vi "test Basic Error Resolution.vi"(8 "error in (no error)":errorcluster, 11 "TestCase in":refnum<class "Task Tests.lvclass">) -> (0 "error out":errorcluster, 3 "TestCase out":refnum<class "Task Tests.lvclass">)   [LabVIEW 2017, in "Task Tests.lvclass"]
uses:
  Task Tests.lvclass
  <vilib>/Utility/error.llb/Error Cluster From Error Code.vi
  <vilib>/ErrorRing/Error Ring.xnode
  <vilib>/addons/_JKI Toolkits/VI Tester/TestCase.llb/TestCase.lvclass
  Futures/Task/Task.lvclass
  C:/Program Files (x86)/National Instruments/LabVIEW 2017/vi.lib/addons/_JKI Toolkits/VI Tester/TestCase.llb/TestCase.lvclass
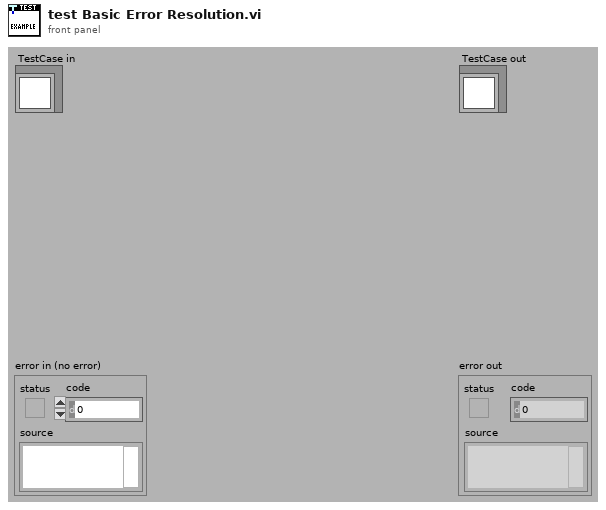
[diagram p1: front panel]
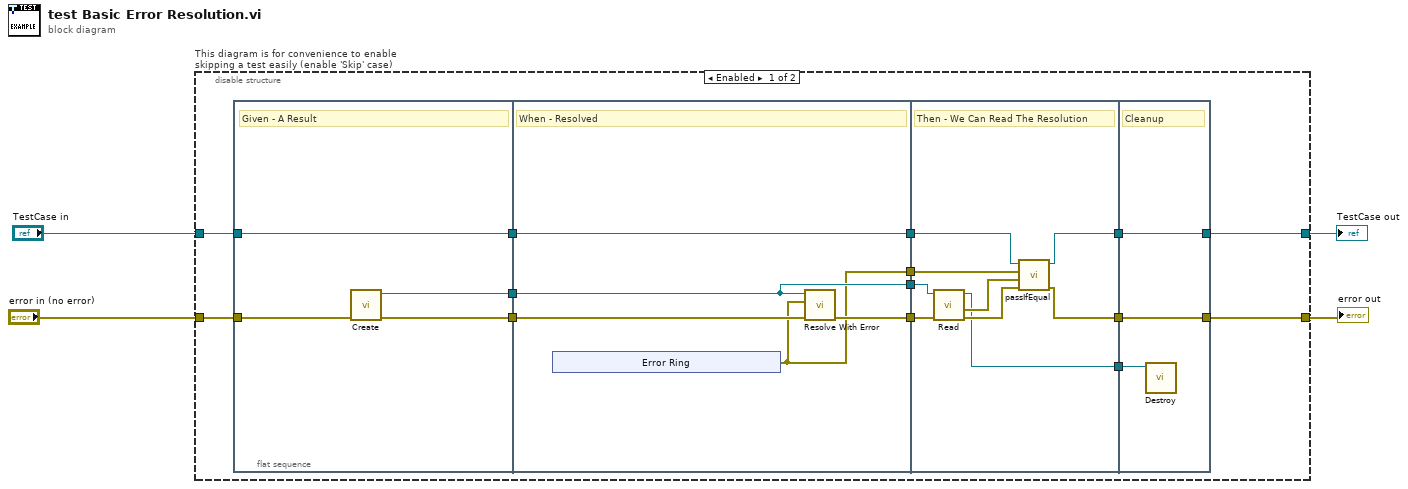
[diagram p0: block diagram]
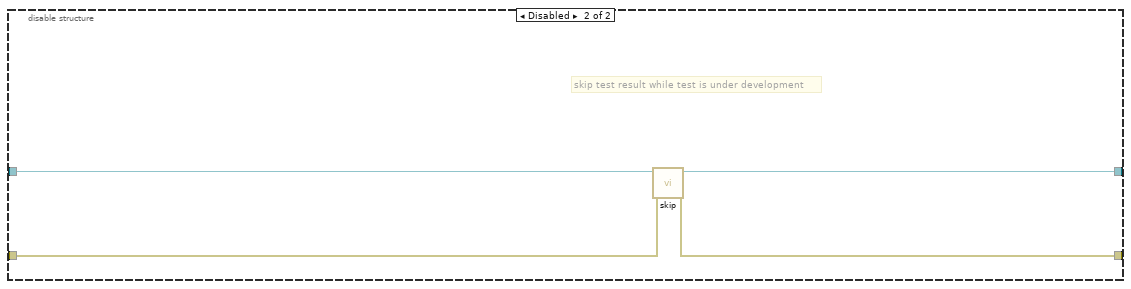
[diagram p2: hidden frame]
diagram:
  n1 = disable-structure "This diagram is for convenience to enable skipping a test easily (enable 'Skip' case)" shown="Enabled" {
    disable-tunnel: "TestCase in" -> [w12 w47]
    disable-tunnel: [w10 w45] -> w1
    disable-tunnel: [w9 w46] -> w3
    disable-tunnel: "error in (no error)" -> [w11 w44]
    frame Enabled {
      n2 = flat-sequence {
        tunnel: w11 -> [w21]
        tunnel: w12 -> [w22]
        tunnel: [w22] -> w18
        tunnel: [w20] -> w17
        tunnel: [w19] -> w8
        tunnel: [w27] -> w16
        tunnel: [w25] -> w15
        tunnel: w18 -> [w27]
        tunnel: w17 -> [w26]
        tunnel: w8 -> [w24]
        tunnel: [w24] -> w7
        tunnel: [w23] -> w6
        tunnel: [w39] -> w14
        tunnel: [w38] -> w13
        tunnel: w16 -> [w40]
        tunnel: w15 -> [w37]
        tunnel: w7 -> [w36]
        tunnel: w6 -> [w35]
        tunnel: [w32] -> w5
        tunnel: [w42] -> w9
        tunnel: [w43] -> w10
        tunnel: w14 -> [w43]
        tunnel: w13 -> [w42]
        tunnel: w5 -> [w41]
        frame #0 {
          # "Given - A Result"
          n3 = call "Create.vi"("error in (no error)"=w21) -> ("error out"=w20:errorcluster, "Result out"=w19:refnum<class "Task.lvclass">)  [unwired: 9 in]
        }
        frame #1 {
          # "When - Resolved"
          n4 = xnode "Error Ring"() -> ("error out"=w23:errorcluster)
          n5 = call "Resolve With Error.vi"("error in (no error)"=w26, "Error"=w23, "Result in"=w24) -> ("error out"=w25:errorcluster)  [unwired: 8 in]
        }
        frame #2 {
          # "Then - We Can Read The Resolution"
          n6 = call "Read.vi"("error in (no error)"=w37, "Result in"=w36) -> ("error out"=w34:errorcluster, "result error"=w33:errorcluster, "Result Out"=w32:refnum<class "Task.lvclass">)  [unwired: 5 in, 2 out]
          n7 = call-dynamic "passIfEqual.vi"("error in (no error)"=w34, "y"=w33, "x"=w35, "TestCase in"=w40) -> ("error out"=w38:errorcluster, "TestCase out"=w39:refnum<class "Task Tests.lvclass">)  [unwired: 6 in]
        }
        frame #3 {
          # "Cleanup"
          n8 = call "Destroy.vi"("Result in"=w41) -> ()  [unwired: 10 in, 1 out]
        }
      }
    }
    frame Disabled {
      # "skip test result while test is under development"
      n9 = call <vilib>:"skip.vi"("error in (no error)"=w44, "TestCase in"=w47) -> ("error out"=w46:errorcluster, "TestCase out"=w45:refnum<class "Task Tests.lvclass">)  [unwired: 8 in]
    }
  }
  "error out" <- w3
  "TestCase out" <- w1
